vi "NAME.vi"(7 "mode":u8, 9 "Name":string="Light", 11 "Python in":string="import machine, utime\n\ntx = machine.Pin('Y9', machine.Pin.OUT)\nrx = machine.Pin('Y10', machine.Pin.IN)\ntx.value(b'\\x00')\nutime.sleep_ms(500)\ntx.value(1)\n\nuart = machine.UART(3)\nuart.init(baudrate=2400, bits=8, parity=None, stop=1)\n\nuart.write(0)\nuart.write(b'\\x40\\x23\\x9C')\n") -> (3 "Python out":string="import machine, utime\n\ntx = machine.Pin('Y9', machine.Pin.OUT)\nrx = machine.Pin('Y10', machine.Pin.IN)\ntx.value(b'\\x00')\nutime.sleep_ms(500)\ntx.value(1)\n\nuart = machine.UART(3)\nuart.init(baudrate=2400, bits=8, parity=None, stop=1)\n\nuart.write(0)\nuart.write(b'\\x40\\x23\\x9C')\nuart.write(b'\\x98\\x00\\x4C\\x69\\x67\\x68\\x74\\x00\\x00\\x00\\x39')\n")   [LabVIEW 2019]
panel:
  out "bytes added":u8[](array[numeric])=[152, 0, 76, 105, 103, 104, 116, 0, 0, 0, 57] format="%.0x"
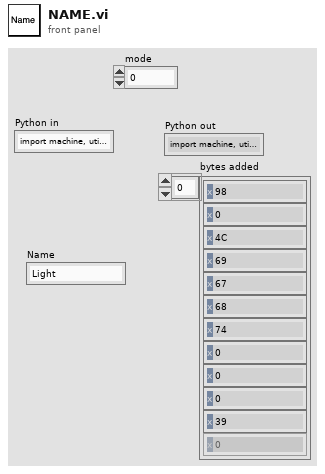
[diagram p1: front panel]
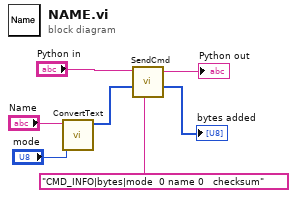
[diagram p0: block diagram]
diagram:
  n1 = call <userlib>:"ConvertText.vi"("mode"="mode", "Name"="Name") -> ("Array"=w4:u8[])  [unwired: 9 in]
  n2 = call <userlib>:"SendCmd.vi"("Comment"="CMD_INFO|bytes|mode  0 name 0   checksum", "Array In"=w4, "Python in"="Python in") -> ("Array Sent"=→"bytes added":u8[], "Python out"=→"Python out":string)  [unwired: 7 in]
